vi "TiePie.Gen.SetOutputEnable.vi"(8 "error in (no error)":errorcluster, 10 "Enable":bool, 11 "GenHandle":T1) -> (0 "error out":errorcluster, 3 "GenHandle out":T1)   [LabVIEW 2013, in "LVTiePie.lvlib"]
uses:
  LVTiePie.lvlib
  TiePie.Gen.handle.ctl
  bin/libtiepie.dll
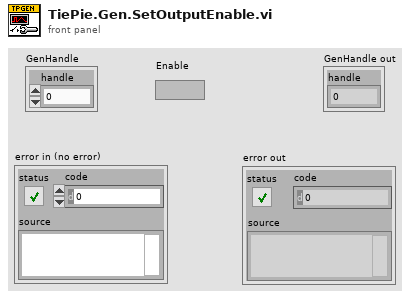
[diagram p1: front panel]
types:
  T1 = typedef "TiePie.Gen.handle.ctl" = cluster{"handle":u32}
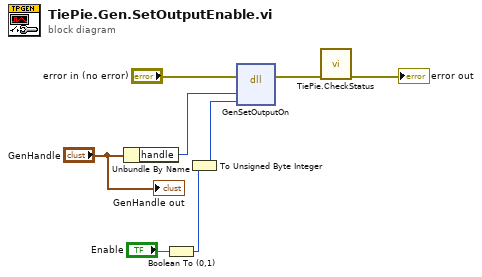
[diagram p0: block diagram]
diagram:
  n1 = Unbundle By Name("GenHandle") -> ("handle"=w7:u32)
  n2 = Boolean To (0,1)(Boolean="Enable") -> (0, 1=w4:i16)
  n3 = To Unsigned Byte Integer(number=w4) -> (unsigned 8bit integer=w3:u8)
  n4 = dll-call lib="D:/Documents and Settings/XP/Moje dokumenty/acas/trunk/support_projects/ACAS_QY/sources/drivers/LVTiePie/bin/libtiepie.dll" fn="GenSetOutputOn"(error in="error in (no error)", "handle"=w7, "enable"=w3) -> (error out=w2:errorcluster)  [unwired: 5 in, 1 out]
  n5 = call "TiePie.CheckStatus.vi"("error in (no error)"=w2) -> ("error out"=→"error out":errorcluster)  [unwired: 10 in]
  "GenHandle out" <- "GenHandle"
